vi "Write Init.vi"(8 "error in (no error)":errorcluster, 10 "Init":bool, 11 "Valve Controller in":refnum<class "Valve Controller.lvclass">) -> (0 "error out":errorcluster, 3 "Valve Controller out":refnum<class "Valve Controller.lvclass">)   [LabVIEW 2011, in "Valve Controller.lvclass"]
uses:
  Valve Controller.lvclass
  Valve Controller.lvclass/Valve Controller.ctl
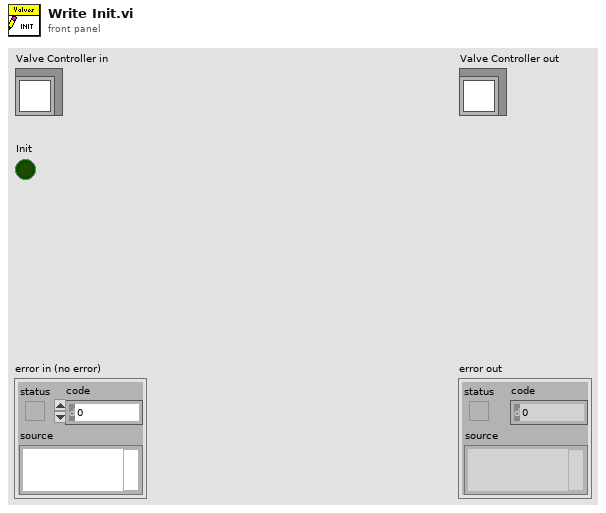
[diagram p1: front panel]
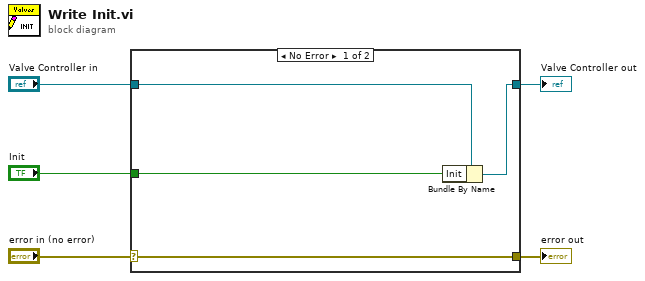
[diagram p0: block diagram]
diagram:
  n1 = case shown="No Error" "error in (no error)" {
    selector: "error in (no error)" -> [w9 w10]
    tunnel: [w9 w10] -> w4
    tunnel: [w7 w11] -> w2
    tunnel: "Valve Controller in" -> [w8 w11]
    tunnel: "Init" -> [w6 _]
    frame No Error {
      n2 = Bundle By Name(cluster=w8, "Init"=w6) -> (w7:refnum<class "Valve Controller.lvclass">)
    }
    frame Error {
    }
  }
  "error out" <- w4
  "Valve Controller out" <- w2
